vi "Insert Data.vi"(7 "Group":string, 8 "error in":errorcluster, 9 "Data":variant, 10 "tag":string, 11 "CVT Session In":T1) -> (0 "error out":errorcluster, 3 "CVT Session Out":T1)   [LabVIEW 2014, in "CVT.lvclass"]
uses:
  CVT.lvclass
  <userlib>/_Session Fwk/Typedefs/Session Handle.ctl
  <userlib>/_Session Fwk/Session - Root.lvclass
  CVT.lvclass/CVT.ctl
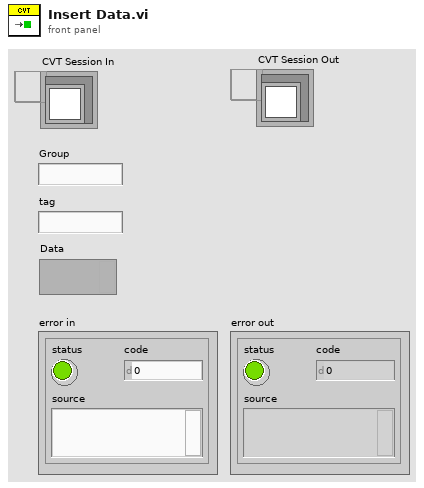
[diagram p1: front panel]
types:
  T1 = typedef "Session - Root.lvclass/Session Handle.ctl" = refnum<data-value>
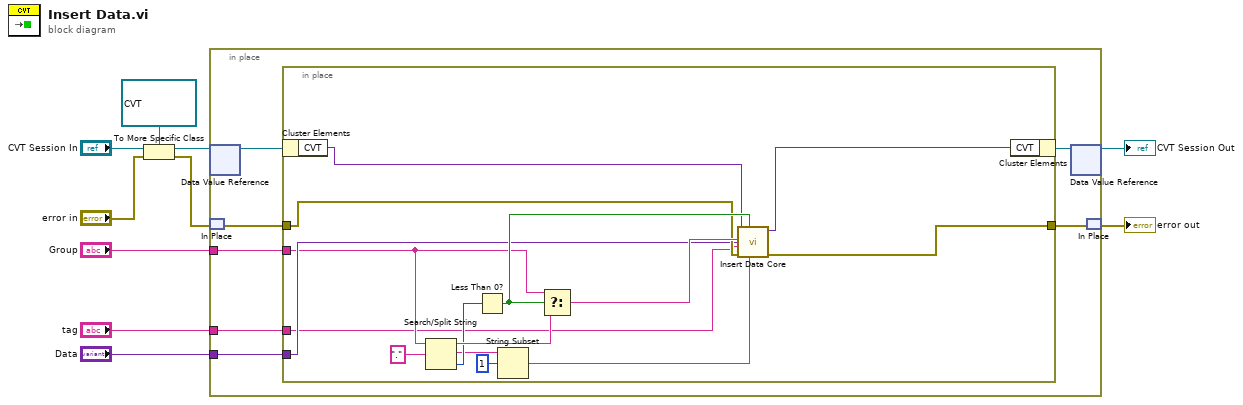
[diagram p0: block diagram]
diagram:
  n1 = To More Specific Class(target class=refnum<data-value> refnum ("CVT Session In"), reference="CVT Session In", error in="error in") -> (specific class reference=w8:refnum<data-value>, error out=w4:errorcluster)
  n2 = in-place {
    in-place-border: "Group" -> [w17]
    in-place-border: "tag" -> [w16]
    in-place-border: "Data" -> [w15]
    n3 = in-place-dvr #1(w8) -> (w14:refnum<class "CVT.lvclass">)  [unwired: 1 out]
    n4 = in-place-match #2(w4) -> (w13:errorcluster)
    n5 = in-place {
      in-place-border: w17 -> [w19]
      in-place-border: w16 -> [w18]
      in-place-border: w15 -> [w20]
      in-place-border: w13 -> [w21]
      in-place-border: [w22] -> w11
      n6 = in-place-cluster #3(w14) -> ("CVT"=w24:variant)
      n7 = Search/Split String(string=w19, search string/char (-)="." ("regular expression")) -> (substring before match=w30:string, match + rest of string=w27:string, offset of match=w29:i32)  [unwired: 1 in]
      n8 = Less Than 0?(x=w29) -> (x < 0?=w31:bool)
      n9 = String Subset(string=w27, offset (0)=1) -> (substring=w25:string)  [unwired: 1 in]
      n10 = Select(t=w19, s=w31, f=w30) -> (s? t:f=w32:string)
      n11 = call "Insert Data Core.vi"("Data"=w20, "Nested Group"=w25, "Nested?"=w31, "error in (no error)"=w21, "tag"=w18, "Group"=w32, "CVT In"=w24) -> ("error out"=w22:errorcluster, "CVT Out"=w23:variant)  [unwired: 2 in]
      n12 = in-place-cluster #3("CVT"=w23) -> (w12:refnum<class "CVT.lvclass">)
    }
    n13 = in-place-dvr #1(w12) -> (→"CVT Session Out":refnum<data-value>)  [unwired: 1 out]
    n14 = in-place-match #2(w11) -> (→"error out":errorcluster)
  }
